vi "getdelaypoints.vi"(1 "delscan_stepsize":dbl caption="stepsize [fs]", 2 "delscan_end":dbl caption="end [fs]", 3 "delscan_start":dbl caption="start [fs]") -> (0 "delaypoints":dbl[](array[numeric]))   [LabVIEW 2020]
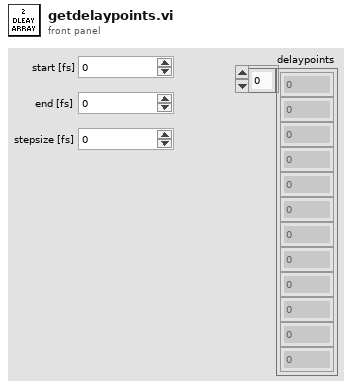
[diagram p1: front panel]
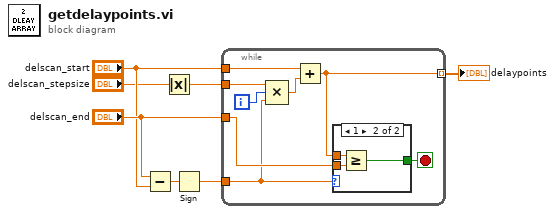
[diagram p0: block diagram]
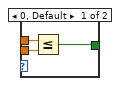
[diagram p2: hidden frame]
diagram:
  n1 = Subtract(x="delscan_end", y="delscan_start") -> (x-y=w4:dbl)
  n2 = Absolute Value(x="delscan_stepsize") -> (abs(x)=w1:dbl)
  n3 = Sign(1:w4) -> (0:w3:dbl)
  n4 = while {
    tunnel: "delscan_start" -> [w15]
    tunnel: w1 -> [w11]
    tunnel: "delscan_end" -> [w12]
    tunnel: [w13] -> w7 mode=indexing
    tunnel: w3 -> [w9]
    i -> [w10]
    stop <- w14 stop-if-true
    n5 = Compound Arithmetic op=MULTIPLY(w11, w10, w9) -> (w8:dbl)
    n6 = Add(x=w15, y=w8) -> (x+y=w13:dbl)
    n7 = case shown="1" w9 {
      tunnel: w13 -> [w17 w21]
      tunnel: w12 -> [w18 w20]
      tunnel: [w16 w19] -> w14
      frame 0, Default {
        n8 = Less Or Equal?(x=w17, y=w18) -> (x <= y?=w16:bool)
      }
      frame 1 {
        n9 = Greater Or Equal?(x=w21, y=w20) -> (x >= y?=w19:bool)
      }
    }
  }
  "delaypoints" <- w7
